vi "SPI_UI.vi"() -> ()   [LabVIEW 2023]
uses:
  ConcreteClasses/ConcreteInstrumentClasses/Multiharp/Multiharp/Types/MH_UIThread_Cmds_T2.ctl
  ConcreteClasses/ConcreteInstrumentClasses/Multiharp/Multiharp/Types/MH_UIThread_Data_T2.ctl
  ConcreteClasses/ConcreteInstrumentClasses/Multiharp/Multiharp/Types/MH_InputChannel.ctl
  ConcreteClasses/ConcreteInstrumentClasses/Multiharp/Multiharp/_lib/PQ/MultiHarp/MH_RefSource.ctl
  ConcreteClasses/ConcreteInstrumentClasses/Multiharp/Multiharp/_lib/PQ/MultiHarp/mhlib_x86_x64_AnyThread.llb/MH_DllPath_global.vi
  <vilib>/Utility/error.llb/DialogType.ctl
  <vilib>/ErrorRing/Error Ring.xnode
  <vilib>/Utility/error.llb/Error Cluster From Error Code.vi
  ConcreteClasses/ConcreteInstrumentClasses/Multiharp/Multiharp/_lib/PQ/MultiHarp/MH_LibVersion_global.vi
  ConcreteClasses/ConcreteInstrumentClasses/Multiharp/Multiharp/_lib/PQ/MultiHarp/MH_MeasMode.ctl
  ConcreteClasses/ConcreteInstrumentClasses/Multiharp/Multiharp/Types/MH_SetInpChanData.ctl
  ConcreteClasses/ConcreteInstrumentClasses/Multiharp/Multiharp/Types/MH_SetInpChanCmds.ctl
  <vilib>/ActorFramework/Message Enqueuer/Message Enqueuer.lvclass
  ConcreteClasses/ConcreteInstrumentClasses/Multiharp/Multiharp/_lib/PQ/MultiHarp/MH_InitInfo.ctl
  typedefs/typedefs.lvlib
panel:
  in  "Init Multiharp":bool
  in  "Refresh(ms)":u32=500
  out "Waveform Chart":dbl[][](graph)
  in  "Monitor Range":i32=40
  in  "Path":path
  in  "FileName 2":string
  in  "Number of Acquisitions":i32=1 min=1 step=1
  out "x*y":dbl
  out "HistoGraph":T1(graph)={0.0, "Resolution"=0.08, "Histograms"=[]}
  in  "Run continuously":enum32{"Running Mode", "Item 1"}(radio) caption="Acquisition"
  in  "Start":bool
  in  "Scale":enum32{"Item 0", "Item 1"}(radio)
  out "CountRates":i32[](graph)
  in  "AllChannels":T2={"Enable"=TRUE, "Offset"=0, "Level"=20, "Edge"=0, "DeadTime"=1000, "UseDeadTime"=FALSE, "SetEnableAllChan"=TRUE, "SetEdgeAllChan"=TRUE, "SetLevelAllChan"=TRUE, "SetOffsetAllChan"=TRUE, "SetUseDTAllChan"=TRUE, "SetDeadTAllChan"=TRUE} {"DeadTime" min=800 max=160000 step=1; "Edge" items=["falling", "rising"]; "Offset" min=-100000 max=100000 step=10; "Level" min=-1200 max=1200 step=1}
  in  "HistoLength":i32(ring)=6 caption="Num Bins" items=["1024", "2048", "4096", "8192", "16384", "32768", "65536"]
  in  "OvlLevel":u32=4294967295 caption="Ovl.Level" min=1 step=1
  in  "StopOvl.":bool=TRUE
  in  "AcqTime":i32=1000 caption="Acqu.           ms" min=1 max=3600000 step=1
  in  "Binning":i32(ring) caption="Resol.            ps" items=["10", "20", "40", "80", "160", "320", "640", "1280", "2560", "5120", "10240", "20480", "40960", "81920", "163840", "327680", "655360", "1310720", "2621440", "5242880", "10485760", "20971520", "41943040"]
  in  "HistoOffset":i32 caption="Offset            ns" min=0 max=100000000 step=1
  in  "Acquire":bool
  in  "stop":bool
  in  "SyncDeadTime":i32=1000 caption="Dead T.   ps" min=800 max=160000 step=1
  in  "UseDeadTime":bool caption="Use DT."
  in  "SyncEdge":i32(ring) caption="Edge" items=["falling", "rising"]
  in  "SyncDivider":i32(ring) caption="Divider" items=["1", "2", "4", "8", "16"]
  in  "SyncOffset":i32 caption="Offset      ps" min=-100000 max=100000 step=10
  in  "SyncLevel":i32=-100 caption="Level      mV" min=-1200 max=1200 step=1
  in  "Channels":T3[](array[typedef])=[{"Name"="Inp.Chan 1", "Enable"=TRUE, "Edge"=0, "Level"=-100, "Offset"=0, "UseDeadTime"=FALSE, "DeadTime"=1000}, {"Name"="Inp.Chan 2", "Enable"=TRUE, "Edge"=0, "Level"=-100, "Offset"=0, "UseDeadTime"=FALSE, "DeadTime"=1000}, {"Name"="Inp.Chan 3", "Enable"=TRUE, "Edge"=0, "Level"=-100, "Offset"=0, "UseDeadTime"=FALSE, "DeadTime"=1000}, {"Name"="Inp.Chan 4", "Enable"=TRUE, "Edge"=0, "Level"=-100, "Offset"=0, "UseDeadTime"=FALSE, "DeadTime"=1000}, {"Name"="Inp.Chan 5", "Enable"=TRUE, "Edge"=0, "Level"=-100, "Offset"=0, "UseDeadTime"=FALSE, "DeadTime"=1000}, {"Name"="Inp.Chan 6", "Enable"=TRUE, "Edge"=0, "Level"=-100, "Offset"=0, "UseDeadTime"=FALSE, "DeadTime"=1000}, {"Name"="Inp.Chan 7", "Enable"=TRUE, "Edge"=0, "Level"=-100, "Offset"=0, "UseDeadTime"=FALSE, "DeadTime"=1000}, {"Name"="Inp.Chan 8", "Enable"=TRUE, "Edge"=0, "Level"=-100, "Offset"=0, "UseDeadTime"=FALSE, "DeadTime"=1000}, {"Name"="Inp.Chan 9", "Enable"=TRUE, "Edge"=0, "Level"=-100, "Offset"=0, "UseDeadTime"=FALSE, "DeadTime"=1000}, {"Name"="Inp.Chan 10", "Enable"=TRUE, "Edge"=0, "Level"=-100, "Offset"=0, "UseDeadTime"=FALSE, "DeadTime"=1000}, {"Name"="Inp.Chan 11", "Enable"=TRUE, "Edge"=0, "Level"=-100, "Offset"=0, "UseDeadTime"=FALSE, "DeadTime"=1000}, {"Name"="Inp.Chan 12", "Enable"=TRUE, "Edge"=0, "Level"=-100, "Offset"=0, "UseDeadTime"=FALSE, "DeadTime"=1000}, {"Name"="Inp.Chan 13", "Enable"=TRUE, "Edge"=0, "Level"=-100, "Offset"=0, "UseDeadTime"=FALSE, "DeadTime"=1000}, {"Name"="Inp.Chan 14", "Enable"=TRUE, "Edge"=0, "Level"=-100, "Offset"=0, "UseDeadTime"=FALSE, "DeadTime"=1000}, {"Name"="Inp.Chan 15", "Enable"=TRUE, "Edge"=0, "Level"=-100, "Offset"=0, "UseDeadTime"=FALSE, "DeadTime"=1000}, {"Name"="Inp.Chan 16", "Enable"=TRUE, "Edge"=0, "Level"=-100, "Offset"=0, "UseDeadTime"=FALSE, "DeadTime"=1000}] {"DeadTime" min=800 max=160000 step=1; "Edge" items=["falling", "rising"]; "Offset" min=-100000 max=100000 step=10; "Level" min=-1200 max=1200 step=1}
  out "SyncRate":string="Sync Rate: 4999950 cps\n"
  out "OverFlow":bool caption="Overflow:"
  out "Status":string="Readout Rate: 8.6 Hz\t\tTotal Counts:\t\tCh. 1: 0 cnts.\t\tCh. 2: 1962112 cnts.\t\tCh. 3: 0 cnts.\t\tCh. 4: 1962112 cnts.\t\tCh. 5: 0 cnts.\t\tCh. 6: 1962112 cnts.\t\tCh. 7: 0 cnts.\t\tCh. 8: 1962112 cnts.\t\tCh. 9: 1962113 cnts.\t\tCh.10: 0 cnts.\t\tCh.11: 1962113 cnts.\t\tCh.12: 0 cnts.\t\tCh.13: 1962113 cnts.\t\tCh.14: 0 cnts.\t\tCh.15: 1962113 cnts.\t\tCh.16: 1962113 cnts.\t\t"
  # "Single Counts"
  # "Coincidences vs time"
  # "Coincidences vs delay"
  # "Acquisition Options"
  # "Acquire Data"
  # "Piezo"
  # "Stage piezo"
  # "Scan"
  # "Jog"
  # "All Channels"
  # "Sync"
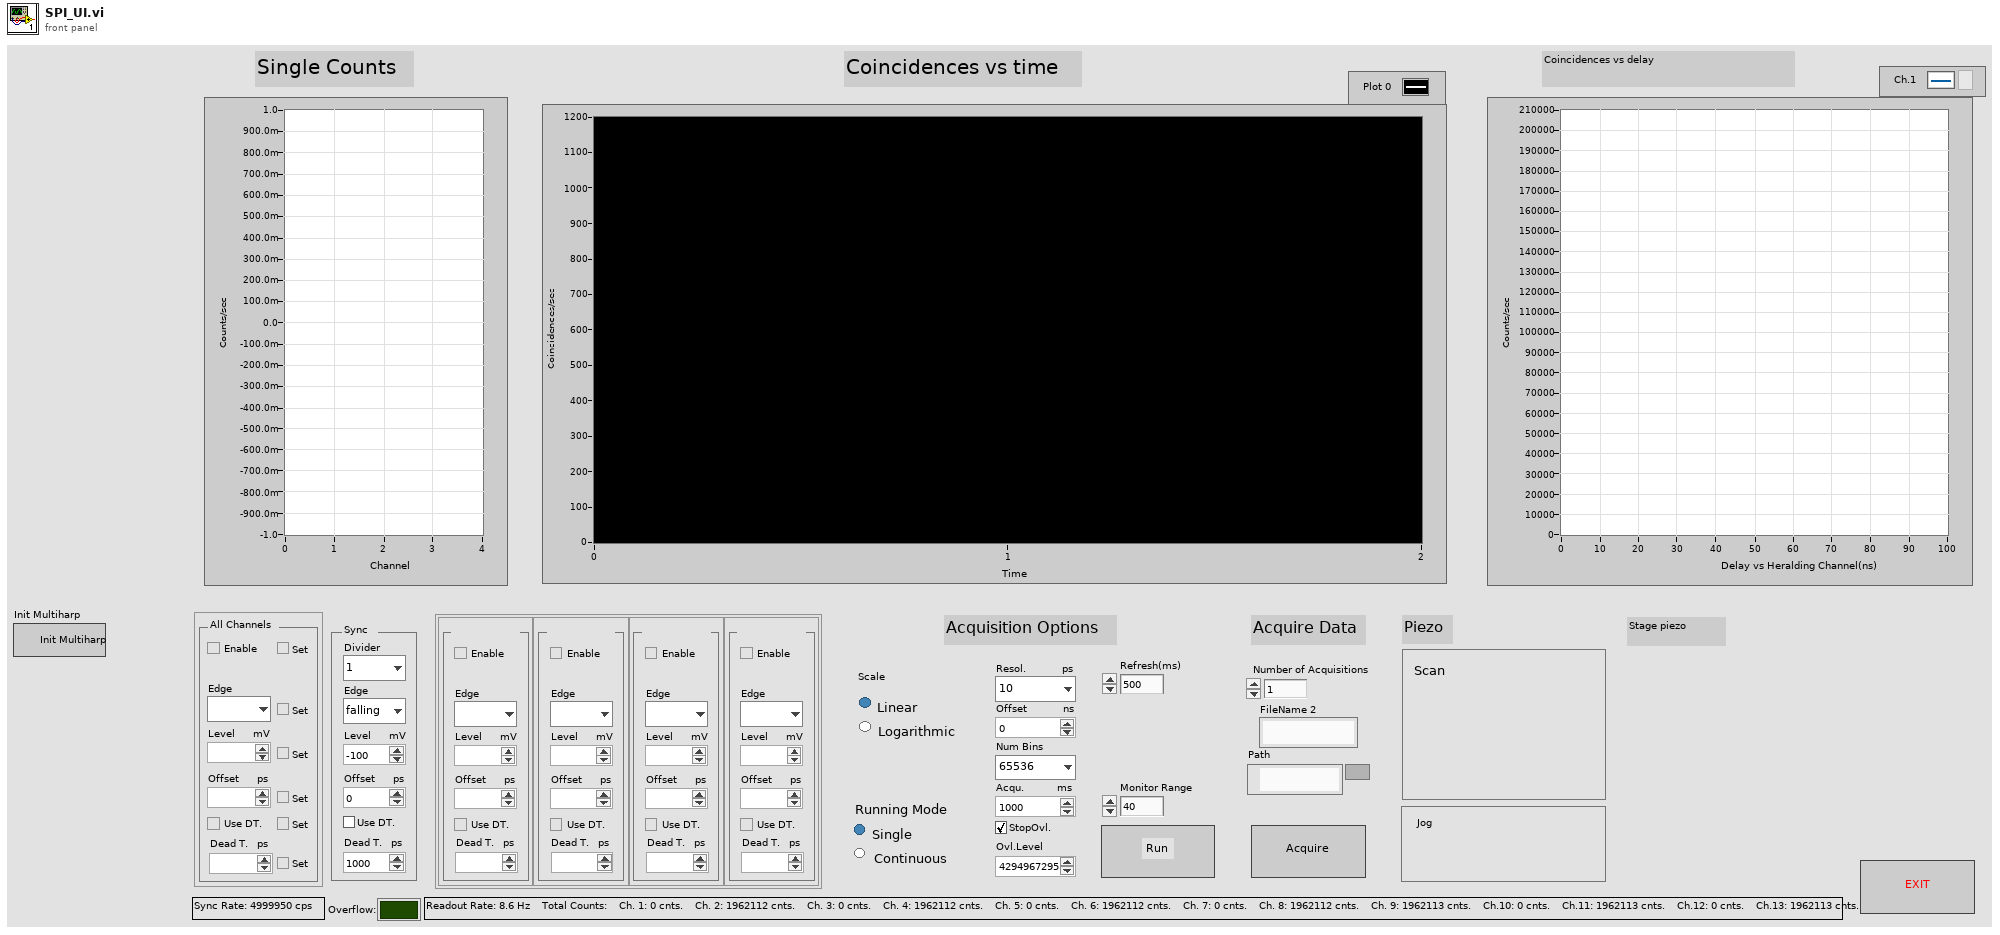
[diagram p1: front panel]
types:
  T1 = cluster{dbl, "Resolution":dbl, "Histograms":u32[][]}
  T2 = cluster{"Enable":bool, "Offset":i32, "Level":i32, "Edge":i32, "DeadTime":i32, "UseDeadTime":bool, "SetEnableAllChan":bool, "SetEdgeAllChan":bool, "SetLevelAllChan":bool, "SetOffsetAllChan":bool, "SetUseDTAllChan":bool, "SetDeadTAllChan":bool}
  T3 = typedef "MH_InputChannel.ctl" = cluster{"Name":string, "Enable":bool, "Edge":i32, "Level":i32, "Offset":i32, "UseDeadTime":bool, "DeadTime":i32}
  T4 = typedef "MH_UIThread_Data_T2.ctl" = cluster{"Init Info":T5, "DevIdx":i32, "SyncDivider":i32, "SyncOffset":i32, "SyncLevel":i32, "Channels":T3[], "CurrentChannels":i32[], "AcqTime":i32, "Binning":i32, "HistoOffset":i32, "HistoLen":i32, "StopOvl.":bool, "OvlLevel":u32, "SyncEdge":i32, "StartMeas":bool, "HistoLength":i32, "Resolution":dbl, "Run cont.":bool, "Status":string, "SyncRate":i32, "BitShift":i32, "HistoAcqTime":dbl, "SyncRateStart":i32, "UseDeadTime":bool, "SyncDeadTime":i32, "SetInpChan":T6[], "max value":u32[], "CoincidenceArray":dbl[][], "Instr Enqueuers":cluster{"MH Enqueuer":refnum<class "Message Enqueuer.lvclass">, "KIM Enqueuer":refnum<class "Message Enqueuer.lvclass">}, "Histo On":bool}
  T5 = typedef "typedefs.lvlib/MH_InitInfo.ctl" = cluster{"Library Version":string, "Serial No.":string, "Model":string, "Partnum":string, "Version":string, "features":i32, "nchannels":i32, "Base Resolution":dbl, "Bin Steps":i32}
  T6 = typedef "MH_SetInpChanData.ctl" = cluster{"Channel":i32, "Cmds":T7[], "Changed":cluster{"Name":bool, "Enable":bool, "Edge":bool, "Level":bool, "Offset":bool, "UseDeadTime":bool, "DeadTime":bool}}
  T7 = typedef "MH_SetInpChanCmds.ctl" = enum16{"SetInpChanEnable", "SetInpChanOffset", "SetInpChanDeadTime", "SetInpChanTrg"}
  T8 = typedef "MH_UIThread_Cmds_T2.ctl" = enum16{"Idle", "Init", "SetInpChan", "SetSyncDivider", "SetSyncTrg", "SetSyncOffset", "SetSyncDeadTime", "SetBinning", "SetHistoOffset", "SetHistoLen", "SetStopOvl", "SetBitShift", "SetHistoAcqTime", "GetRates", "GetAllRates", "StartMeas", "StopMeas", "AbortMeas", "GetResolution", "GetHistos", "GetAllHistos", "ReadFiFo", "WriteStatus", "Resize", "EnableControls", "DisableControls", "Error", "Exit", "Acquire", "InitAcquisition"}
  T9 = enum8{"Enabled", "Disabled", "Disabled and Grayed Out"}
  T10 = typedef "MH_InputChannel2.ctl" = cluster{"Name":string, "Enable":bool, "Edge":i32, "Level":i32, "Offset":i32, "UseDeadTime":bool, "DeadTime":i32}
  T11 = cluster{"[0]":bool, "[1]":bool, "[2]":bool, "[3]":bool, "[4]":bool, "[5]":bool}
  T12 = typedef "MH_MeasMode.ctl" = i32
  T13 = typedef "MH_RefSource.ctl" = enum16{"INTERNAL", "EXTERNAL_10MHZ", "WR_MASTER_GENERIC", "WR_SLAVE_GENERIC", "WR_GRANDM_GENERIC", "EXTN_GPS_PPS", "EXTN_GPS_PPS_UART", "WR_MASTER_MHARP", "WR_SLAVE_MHARP", "WR_GRANDM_MHARP"}
  T14 = cluster{dbl, "Resolution":dbl, "Histogram":u32[][]}
  T15 = typedef "DialogType.ctl" = u16
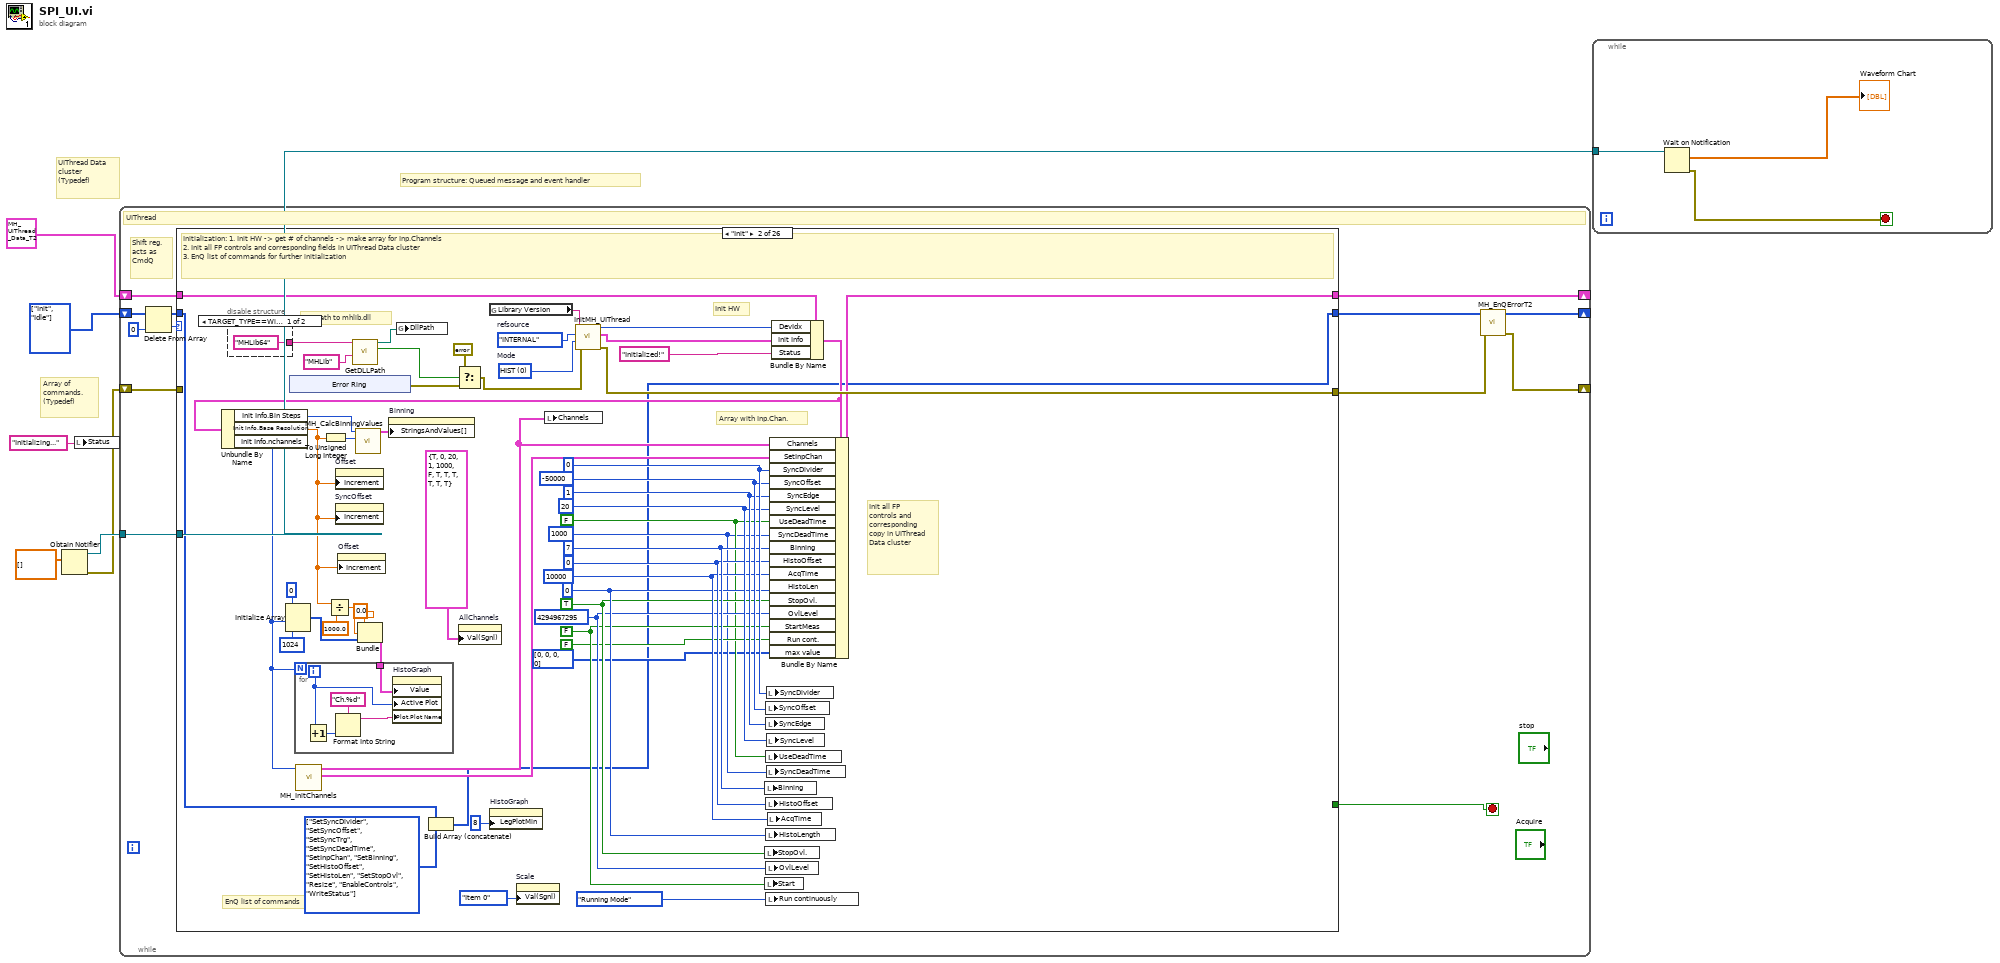
[diagram p0: block diagram]
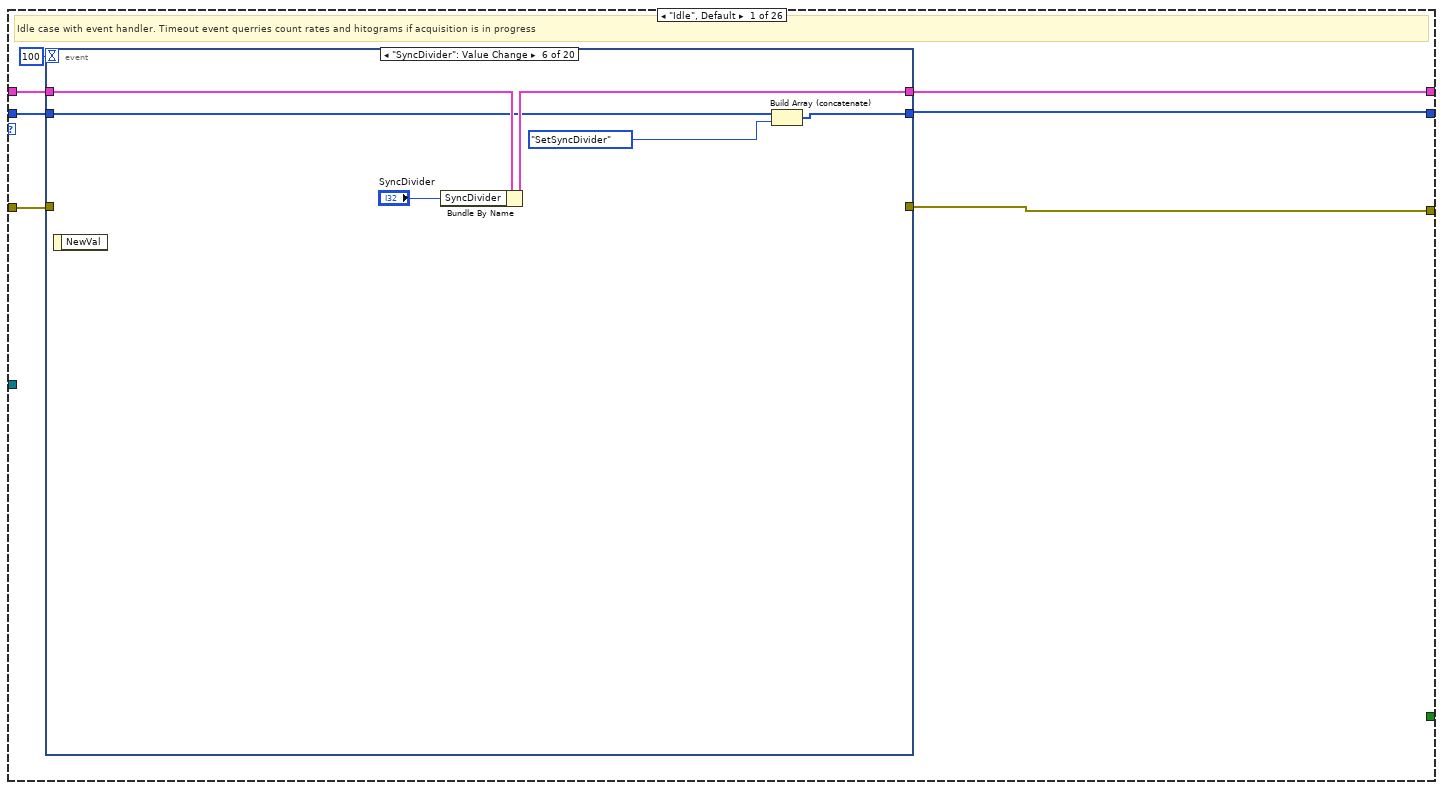
[diagram p2: hidden frame]
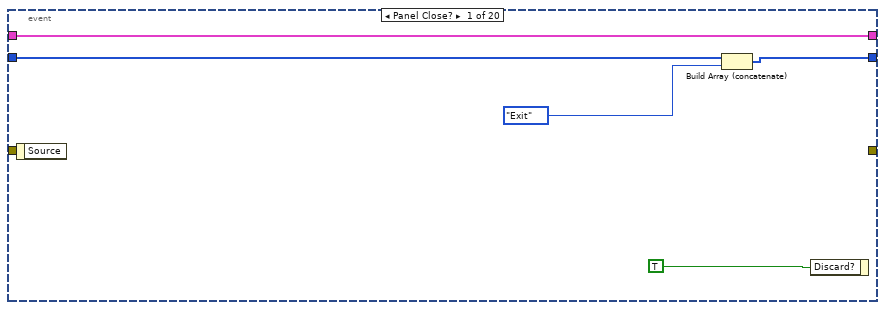
[diagram p3: hidden frame]
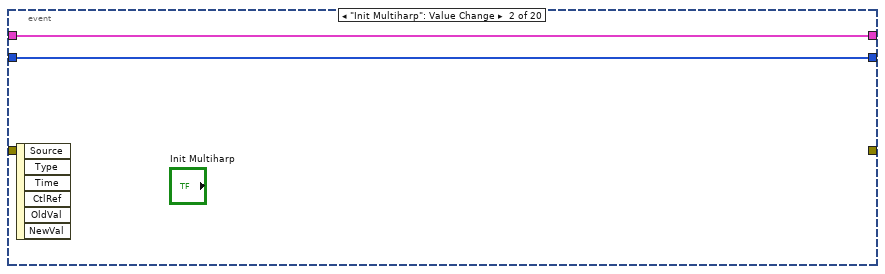
[diagram p4: hidden frame]
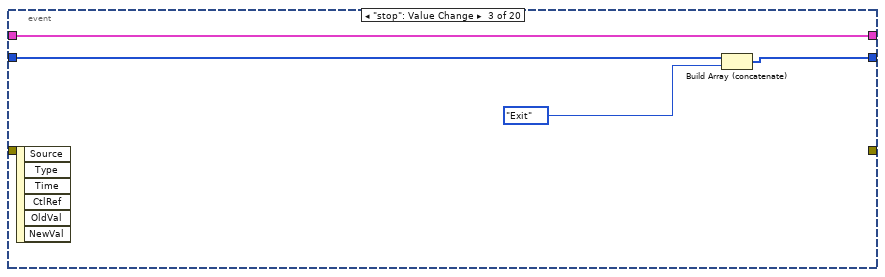
[diagram p5: hidden frame]
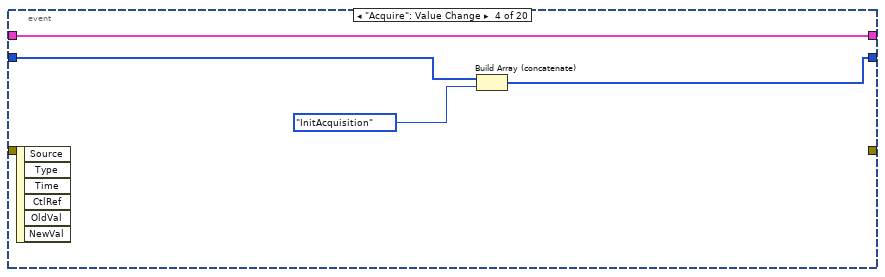
[diagram p6: hidden frame]
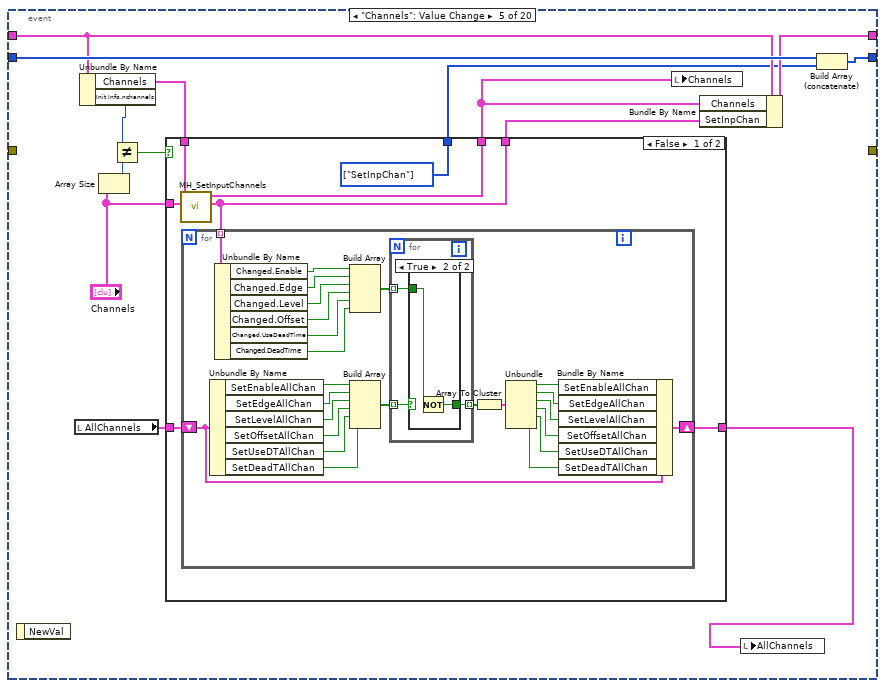
[diagram p7: hidden frame]
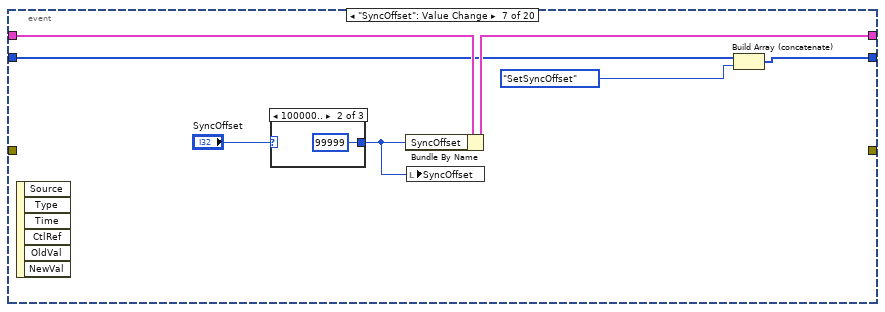
[diagram p10: hidden frame]
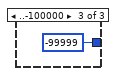
[diagram p12: hidden frame]
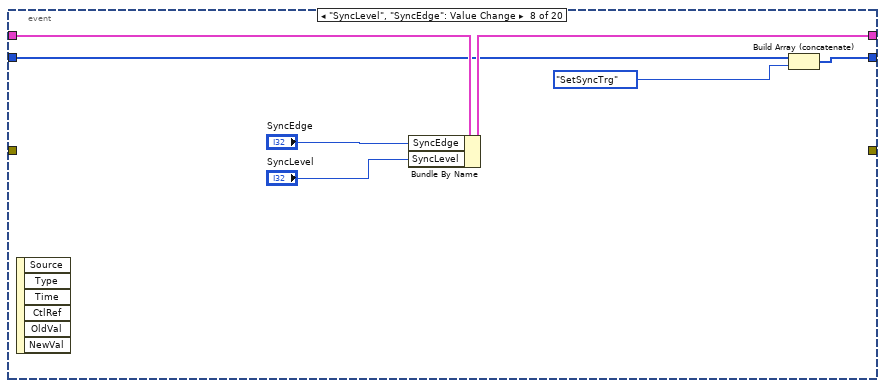
[diagram p13: hidden frame]
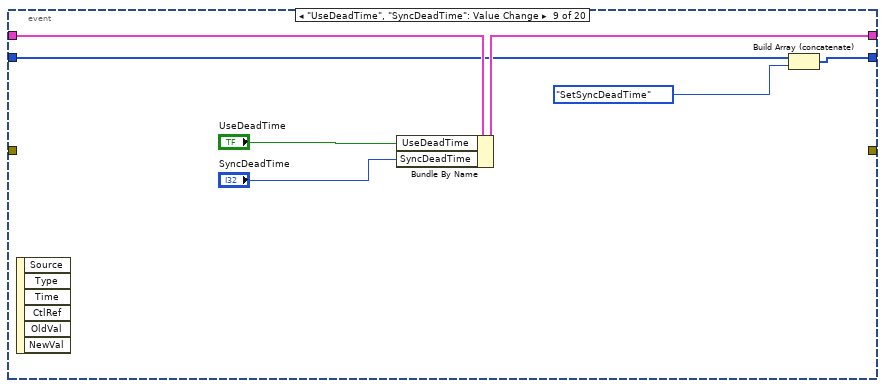
[diagram p14: hidden frame]
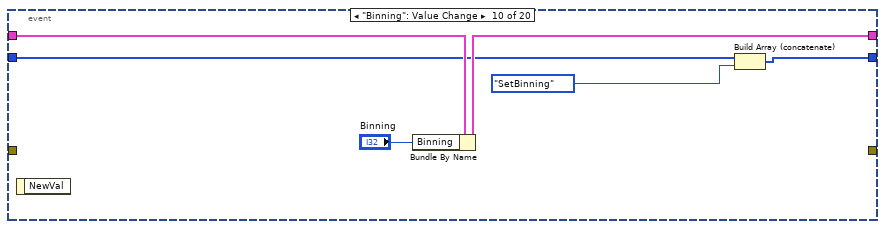
[diagram p15: hidden frame]
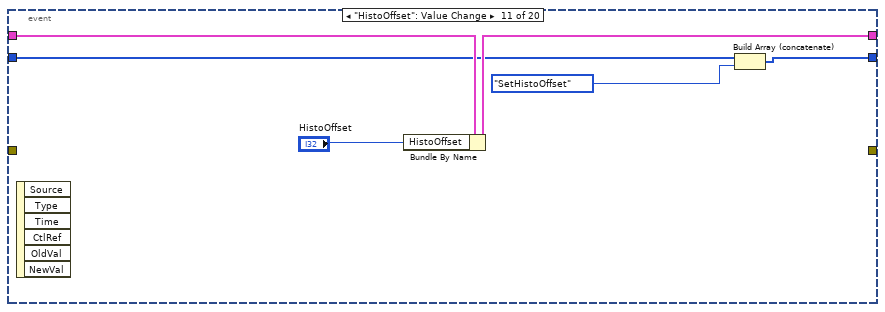
[diagram p16: hidden frame]
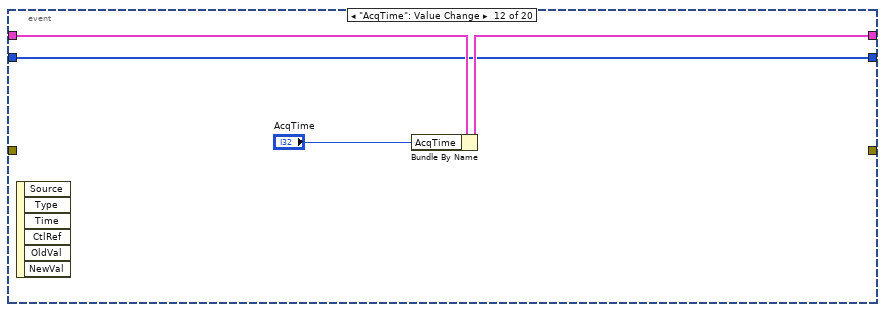
[diagram p17: hidden frame]
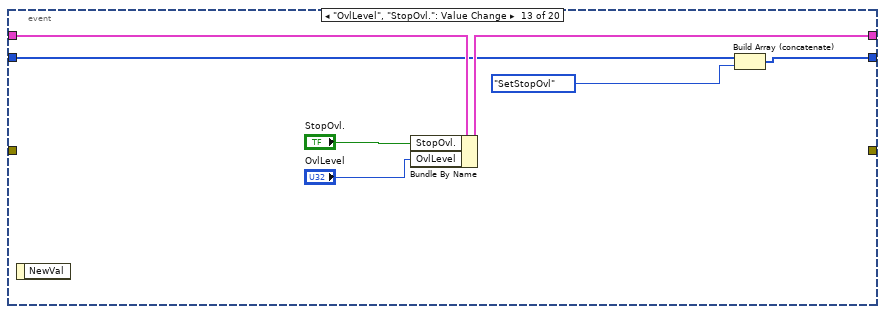
[diagram p18: hidden frame]
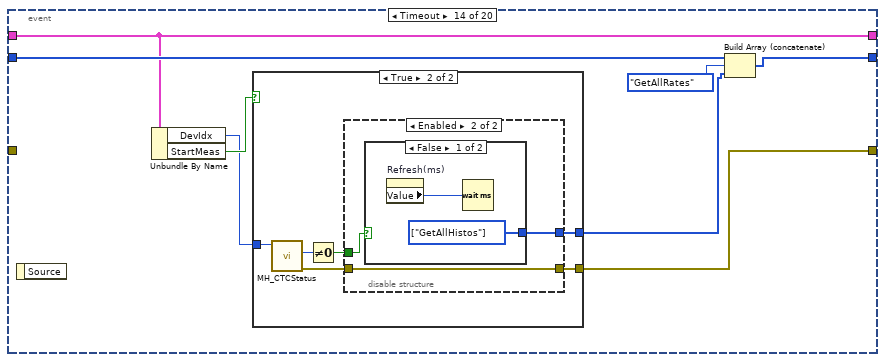
[diagram p19: hidden frame]
diagram:
  w6 = T8[] [enum."Init", enum."Idle"] items=["Idle", "Init", "SetInpChan", "SetSyncDivider", "SetSyncTrg", "SetSyncOffset", "SetSyncDeadTime", "SetBinning", "SetHistoOffset", "SetHistoLen", "SetStopOvl", "SetBitShift", "SetHistoAcqTime", "GetRates", "GetAllRates", "StartMeas", "StopMeas", "AbortMeas", "GetResolution", "GetHistos", "GetAllHistos", "ReadFiFo", "WriteStatus", "Resize", "EnableControls", "DisableControls", "Error", "Exit", "Acquire", "InitAcquisition"]
  # "Array of commands.\n(Typedef)"
  # "Program structure: Queued message and event handler"
  # "UIThread Data cluster\n(Typedef)"
  n1 = Obtain Notifier(notification data type=dbl[][] [] ("element data type")) -> (notifier out=w2:refnum<notifier>, error out=w1:errorcluster)  [unwired: 3 in, 1 out]
  n2 = local write "Status"("Initializing..." ("Status")) -> ()
  n3 = while {
    shift-right: [w9] -> _
    shift-left: w6 -> [w15]
    shift-right: [w18] -> _
    shift-left: T4 {"Init Info"={"Library Version"="", "Serial No."="", "Model"="", "Partnum"="", "Version"="", "features"=0, "nchannels"=0, "Base Resolution"=0.0, "Bin Steps"=0}, "DevIdx"=0, "SyncDivider"=1, "SyncOffset"=0, "SyncLevel"=50, "Channels"=[], "CurrentChannels"=[], "AcqTime"=1, "Binning"=1, "HistoOffset"=1, "HistoLen"=1024, "StopOvl."=FALSE, "OvlLevel"=1024, "SyncEdge"=10, "StartMeas"=FALSE, "HistoLength"=0, "Resolution"=0.0, "Run cont."=FALSE, "Status"="", "SyncRate"=0, "BitShift"=0, "HistoAcqTime"=0.0, "SyncRateStart"=0, "UseDeadTime"=FALSE, "SyncDeadTime"=800, "SetInpChan"=[], "max value"=[], "CoincidenceArray"=[], "Instr Enqueuers"={"MH Enqueuer"=refnum, "KIM Enqueuer"=refnum}, "Histo On"=FALSE} -> [w17]
    shift-right: [w10] -> _
    shift-left: w1 -> [w16]
    tunnel: w2 -> [w8]
    stop <- w19 stop-if-true
    # "Shift reg.\nacts as\nCmdQ"
    # "UIThread"
    n4 = Delete From Array(array=w15, index=0) -> (deleted portion=w13:T8, array with subset deleted=w12:T8[])  [unwired: 1 in]
    n5 = case shown="\"Init\"" w13 {
      tunnel: [_ _ _ _ _ _ _ _ _ _ _ _ _ _ _ _ _ _ _ _ _ _ _ TRUE _ _] -> w19
      tunnel: [w26 w291 w331 w335 w349 w361 w370 w377 w382 w385 w395 w406 w417 w433 w445 w459 w467 w487 w552 w576 w583 w595 w602 w612 w615 w625] -> w18
      tunnel: w17 -> [w25 w296 w331 w335 w349 w361 w370 w377 w382 w386 w395 w406 w417 w434 w446 w460 w468 w488 w552 w576 w583 w595 w602 w612 w615 w625]
      tunnel: [w22 w312 w333 w334 w348 w360 w369 w376 w381 w389 w394 w402 w416 w440 w448 w462 w469 w485 w548 _ _ _ _ w607 w616 w626] -> w11
      tunnel: w16 -> [w20 _ _ _ _ _ _ _ _ _ _ _ _ _ _ _ _ _ _ _ _ _ w603 w610 _ _]
      tunnel: w12 -> [w24 w311 w332 w341 w344 w350 w366 w373 w378 w383 w390 w396 w407 w436 w443 w457 w463 w471 w528 w574 w577 w589 _ w605 w622 w628]
      tunnel: w8 -> [_ _ _ _ _ _ _ _ _ _ _ _ _ _ _ _ _ w482 _ _ _ _ _ w606 _ _]
      tunnel: [w21 w262 w332 w341 w344 w350 w366 w371 w378 w383 w390 w396 w407 w431 w441 w455 w463 w471 w528 w574 w577 w589 w601 w605 w614 w624] -> w7
      frame "Idle", Default {
        # "Idle case with event handler. Timeout event querries count rates and hitograms if acquisition is in progress"
        n6 = event shown="[5] \"SyncDivider\": Value Change" {
          selector: _ -> [_ _ _ _ _ _ _ _ _ _ _ _ _ _ _ _ _ _ _ _]
          dyn-events: _ -> [_ _ _ _ _ _ _ _ _ _ _ _ _ _ _ _ _ _ _ _]
          timeout: 100 -> [_ _ _ _ _ _ _ _ _ _ _ _ _ _ _ _ _ _ _ _]
          tunnel: [w27 w33 w34 w38 w42 w96 w102 w112 w119 w126 w132 w138 w142 w153 w174 w180 w188 w195 w198 w202] -> w21
          tunnel: [w30 w32 w37 w41 w48 w100 w107 w117 w124 w130 w136 w140 w147 w155 w178 w182 w193 w197 w201 w206] -> w26
          tunnel: w25 -> [w30 w32 w37 w41 w50 w101 w108 w118 w125 w131 w137 w141 w148 w155 w179 w183 w194 w197 w201 w207]
          tunnel: w24 -> [w29 w33 w36 w40 w55 w98 w106 w115 w123 w129 w135 w138 w146 w156 w177 w185 w188 w195 w199 w212]
          tunnel: [_ _ _ _ _ _ _ _ _ _ _ _ _ w154 _ _ _ _ _ _] -> w22
          tunnel: w20 -> [_ _ _ _ _ _ _ _ _ _ _ _ _ _ _ _ _ _ _ _]
          event Panel Close? {
            n7 = event-data() -> ()  [unwired: 1 in, 1 out]
            n8 = Build Array (concatenate)(w29, MH_UIThread_Cmds_T2."Exit") -> (w27:T8[])
            n9 = event-data("Discard?"=TRUE) -> ()  [unwired: 1 in, 1 out]
          }
          event "Init Multiharp": Value Change {
            n10 = event-data() -> ()  [unwired: 1 in, 6 out]
          }
          event "stop": Value Change {
            n11 = event-data() -> ()  [unwired: 1 in, 6 out]
            n12 = Build Array (concatenate)(w36, MH_UIThread_Cmds_T2."Exit") -> (w34:T8[])
          }
          event "Acquire": Value Change {
            n13 = event-data() -> ()  [unwired: 1 in, 6 out]
            n14 = Build Array (concatenate)(w40, MH_UIThread_Cmds_T2."InitAcquisition") -> (w38:T8[])
          }
          event "Channels": Value Change {
            n15 = event-data() -> ()  [unwired: 1 in, 1 out]
            n16 = local read "AllChannels"() -> (w44:T2)
            n17 = Unbundle By Name(w50) -> ("Channels"=w51:T3[], "Init Info.nchannels"=w54:i32)
            n18 = Array Size(array="Channels") -> (size(s)=w53:i32)
            n19 = Not Equal?(x=w54, y=w53) -> (x != y?=w52:bool)
            n20 = case shown="False" w52 {
              tunnel: "Channels" -> [w61 _]
              tunnel: [w60 w95] -> w49
              tunnel: w51 -> [w62 w95]
              tunnel: [w58 _] -> w47
              tunnel: [w59 _] -> w45
              tunnel: w44 -> [w57 w94]
              tunnel: [w56 w94] -> w43
              frame False {
                w59 = T8[] [enum."SetInpChan"] items=["Idle", "Init", "SetInpChan", "SetSyncDivider", "SetSyncTrg", "SetSyncOffset", "SetSyncDeadTime", "SetBinning", "SetHistoOffset", "SetHistoLen", "SetStopOvl", "SetBitShift", "SetHistoAcqTime", "GetRates", "GetAllRates", "StartMeas", "StopMeas", "AbortMeas", "GetResolution", "GetHistos", "GetAllHistos", "ReadFiFo", "WriteStatus", "Resize", "EnableControls", "DisableControls", "Error", "Exit", "Acquire", "InitAcquisition"] ("array")
                n21 = call "MH_SetInputChannels.vi"("Channels new"=w61, "Channels old"=w62) -> ("SetInpChan"=w58:T6[], "Channels"=w60:T10[])  [unwired: 8 in]
                n22 = for {
                  tunnel: w58 -> [w87] mode=indexing
                  shift-right: [w69] -> w56
                  shift-left: w57 -> [w71]
                  n23 = Unbundle By Name(w71) -> ("SetEnableAllChan"=w80:bool, "SetEdgeAllChan"=w79:bool, "SetLevelAllChan"=w78:bool, "SetOffsetAllChan"=w77:bool, "SetUseDTAllChan"=w76:bool, "SetDeadTAllChan"=w75:bool)
                  n24 = Unbundle By Name(w87) -> ("Changed.Enable"=w86:bool, "Changed.Edge"=w85:bool, "Changed.Level"=w84:bool, "Changed.Offset"=w83:bool, "Changed.UseDeadTime"=w82:bool, "Changed.DeadTime"=w81:bool)
                  n25 = Build Array(w86, w85, w84, w83, w82, w81) -> (w73:bool[])
                  n26 = Build Array(w80, w79, w78, w77, w76, w75) -> (w74:bool[])
                  n27 = for {
                    tunnel: w74 -> [w90] mode=indexing
                    tunnel: w73 -> [w88] mode=indexing
                    tunnel: [w89] -> w72 mode=indexing
                    n28 = case shown="True" w90 {
                      selector: w90 -> [w91 _]
                      tunnel: [w91 w92] -> w89
                      tunnel: w88 -> [_ w93]
                      frame False {
                      }
                      frame True {
                        n29 = Not(x=w93) -> (.not. x?=w92:bool)
                      }
                    }
                  }
                  n30 = Array To Cluster(array=w72) -> (cluster=w70:T11)
                  n31 = Unbundle(w70) -> ("[0]"=w68:bool, "[1]"=w67:bool, "[2]"=w66:bool, "[3]"=w65:bool, "[4]"=w64:bool, "[5]"=w63:bool)
                  n32 = Bundle By Name(cluster=w71, "SetEnableAllChan"=w68, "SetEdgeAllChan"=w67, "SetLevelAllChan"=w66, "SetOffsetAllChan"=w65, "SetUseDTAllChan"=w64, "SetDeadTAllChan"=w63) -> (w69:T2)
                }
              }
              frame True {
              }
            }
            n33 = local write "Channels"(w49) -> ()
            n34 = Bundle By Name(cluster=w50, "Channels"=w49, "SetInpChan"=w47) -> (w48:T4)
            n35 = local write "AllChannels"(w43) -> ()
            n36 = Build Array (concatenate)(w55, w45) -> (w42:T8[])
          }
          event "SyncDivider": Value Change {
            n37 = event-data() -> ()  [unwired: 1 in, 1 out]
            n38 = Bundle By Name(cluster=w101, "SyncDivider"="SyncDivider") -> (w100:T4)
            n39 = Build Array (concatenate)(w98, MH_UIThread_Cmds_T2."SetSyncDivider") -> (w96:T8[])
          }
          event "SyncOffset": Value Change {
            n40 = event-data() -> ()  [unwired: 1 in, 6 out]
            n41 = case shown="100000.." "SyncOffset" {
              selector: "SyncOffset" -> [w109 _ _]
              tunnel: [w109 99999 ("SyncOffset") -99999 ("SyncOffset")] -> w103
              frame Default {
              }
              frame 100000.. {
              }
              frame ..-100000 {
              }
            }
            n42 = Bundle By Name(cluster=w108, "SyncOffset"=w103) -> (w107:T4)
            n43 = local write "SyncOffset"(w103) -> ()
            n44 = Build Array (concatenate)(w106, MH_UIThread_Cmds_T2."SetSyncOffset") -> (w102:T8[])
          }
          event "SyncLevel", "SyncEdge": Value Change {
            n45 = event-data() -> ()  [unwired: 1 in, 6 out]
            n46 = Bundle By Name(cluster=w118, "SyncEdge"="SyncEdge", "SyncLevel"="SyncLevel") -> (w117:T4)
            n47 = Build Array (concatenate)(w115, MH_UIThread_Cmds_T2."SetSyncTrg") -> (w112:T8[])
          }
          event "UseDeadTime", "SyncDeadTime": Value Change {
            n48 = event-data() -> ()  [unwired: 1 in, 6 out]
            n49 = Bundle By Name(cluster=w125, "UseDeadTime"="UseDeadTime", "SyncDeadTime"="SyncDeadTime") -> (w124:T4)
            n50 = Build Array (concatenate)(w123, MH_UIThread_Cmds_T2."SetSyncDeadTime") -> (w119:T8[])
          }
          event "Binning": Value Change {
            n51 = event-data() -> ()  [unwired: 1 in, 1 out]
            n52 = Bundle By Name(cluster=w131, "Binning"="Binning") -> (w130:T4)
            n53 = Build Array (concatenate)(w129, MH_UIThread_Cmds_T2."SetBinning") -> (w126:T8[])
          }
          event "HistoOffset": Value Change {
            n54 = event-data() -> ()  [unwired: 1 in, 6 out]
            n55 = Bundle By Name(cluster=w137, "HistoOffset"="HistoOffset") -> (w136:T4)
            n56 = Build Array (concatenate)(w135, MH_UIThread_Cmds_T2."SetHistoOffset") -> (w132:T8[])
          }
          event "AcqTime": Value Change {
            n57 = event-data() -> ()  [unwired: 1 in, 6 out]
            n58 = Bundle By Name(cluster=w141, "AcqTime"="AcqTime") -> (w140:T4)
          }
          event "OvlLevel", "StopOvl.": Value Change {
            n59 = event-data() -> ()  [unwired: 1 in, 1 out]
            n60 = Bundle By Name(cluster=w148, "StopOvl."="StopOvl.", "OvlLevel"="OvlLevel") -> (w147:T4)
            n61 = Build Array (concatenate)(w146, MH_UIThread_Cmds_T2."SetStopOvl") -> (w142:T8[])
          }
          event Timeout {
            n62 = event-data() -> ()  [unwired: 1 in, 1 out]
            n63 = Unbundle By Name(w155) -> ("DevIdx"=w150:i32, "StartMeas"=w151:bool)
            n64 = case shown="True" w151 {
              tunnel: w150 -> [_ w162]
              tunnel: [_ w160] -> w149
              tunnel: [_ w157] -> w154
              frame False {
              }
              frame True {
                n65 = call "MH_CTCStatus.vi"("devidx"=w162) -> ("error out"=w158:errorcluster, "ctcstatus"=w161:i32)  [unwired: 8 in, 1 out]
                n66 = Not Equal To 0?(x=w161) -> (x != 0?=w159:bool)
                n67 = disable-structure shown="Enabled" {
                  disable-tunnel: [w167 w169] -> w160
                  disable-tunnel: w159 -> [w165 w170]
                  disable-tunnel: w158 -> [w163 w168]
                  disable-tunnel: [w163 w168] -> w157
                  frame Disabled {
                    w164 = T8[] [enum."GetAllHistos"] items=["Idle", "Init", "SetInpChan", "SetSyncDivider", "SetSyncTrg", "SetSyncOffset", "SetSyncDeadTime", "SetBinning", "SetHistoOffset", "SetHistoLen", "SetStopOvl", "SetBitShift", "SetHistoAcqTime", "GetRates", "GetAllRates", "StartMeas", "StopMeas", "AbortMeas", "GetResolution", "GetHistos", "GetAllHistos", "ReadFiFo", "WriteStatus", "Resize", "EnableControls", "DisableControls", "Error", "Exit", "Acquire", "InitAcquisition"]
                    w166 = T8[] [enum."StopMeas"] items=["Idle", "Init", "SetInpChan", "SetSyncDivider", "SetSyncTrg", "SetSyncOffset", "SetSyncDeadTime", "SetBinning", "SetHistoOffset", "SetHistoLen", "SetStopOvl", "SetBitShift", "SetHistoAcqTime", "GetRates", "GetAllRates", "StartMeas", "StopMeas", "AbortMeas", "GetResolution", "GetHistos", "GetAllHistos", "ReadFiFo", "WriteStatus", "Resize", "EnableControls", "DisableControls", "Error", "Exit", "Acquire", "InitAcquisition"]
                    n68 = Select(t=w166, s=w165, f=w164) -> (s? t:f=w167:T8[])
                  }
                  frame Enabled {
                    n69 = case shown="False" w170 {
                      tunnel: [w172 w173] -> w169
                      frame False {
                        w172 = T8[] [enum."GetAllHistos"] items=["Idle", "Init", "SetInpChan", "SetSyncDivider", "SetSyncTrg", "SetSyncOffset", "SetSyncDeadTime", "SetBinning", "SetHistoOffset", "SetHistoLen", "SetStopOvl", "SetBitShift", "SetHistoAcqTime", "GetRates", "GetAllRates", "StartMeas", "StopMeas", "AbortMeas", "GetResolution", "GetHistos", "GetAllHistos", "ReadFiFo", "WriteStatus", "Resize", "EnableControls", "DisableControls", "Error", "Exit", "Acquire", "InitAcquisition"]
                        n70 = property on="Refresh(ms)" class="DigNum (strict)"() -> ("Value"=w171:u32)  [unwired: 2 in, 2 out]
                        n71 = Wait (ms)(milliseconds to wait=w171) -> ()  [unwired: 1 out]
                      }
                      frame True {
                        w173 = T8[] [enum."StopMeas"] items=["Idle", "Init", "SetInpChan", "SetSyncDivider", "SetSyncTrg", "SetSyncOffset", "SetSyncDeadTime", "SetBinning", "SetHistoOffset", "SetHistoLen", "SetStopOvl", "SetBitShift", "SetHistoAcqTime", "GetRates", "GetAllRates", "StartMeas", "StopMeas", "AbortMeas", "GetResolution", "GetHistos", "GetAllHistos", "ReadFiFo", "WriteStatus", "Resize", "EnableControls", "DisableControls", "Error", "Exit", "Acquire", "InitAcquisition"]
                      }
                    }
                  }
                }
              }
            }
            n72 = Build Array (concatenate)(w156, MH_UIThread_Cmds_T2."GetAllRates", w149) -> (w153:T8[])
          }
          event "HistoLength": Value Change {
            n73 = event-data() -> ()  [unwired: 1 in, 6 out]
            n74 = Bundle By Name(cluster=w179, "HistoLen"="HistoLength") -> (w178:T4)
            n75 = Build Array (concatenate)(w177, MH_UIThread_Cmds_T2."SetHistoLen") -> (w174:T8[])
          }
          event "Start": Value Change {
            n76 = event-data() -> ()  [unwired: 1 in, 1 out]
            n77 = Select(t=MH_UIThread_Cmds_T2."StartMeas", s="Start", f=MH_UIThread_Cmds_T2."AbortMeas") -> (s? t:f=w184:T8)
            n78 = Bundle By Name(cluster=w183, "StartMeas"="Start") -> (w182:T4)
            n79 = Build Array (concatenate)(w185, w184) -> (w180:T8[])
          }
          event "Run continuously": Value Change {
            n80 = event-data() -> ()  [unwired: 1 in, 1 out]
            n81 = Number To Boolean Array(number="Run continuously") -> (Boolean array=w191:bool[])
            n82 = Delete From Array(array=w191, index=0) -> (deleted portion=w189:bool)  [unwired: 1 in, 1 out]
            n83 = Bundle By Name(cluster=w194, "Run cont."=w189) -> (w193:T4)
          }
          event "Scale": Value Change {
            n84 = event-data() -> ()  [unwired: 1 in, 1 out]
            n85 = property on="HistoGraph" class="WFGraph (strict)"("YScale.Mapping Mode"="Scale") -> ()  [unwired: 2 in, 2 out]
          }
          event Panel Resize {
            n86 = event-data() -> ()  [unwired: 1 in, 1 out]
            n87 = Build Array (concatenate)(w199, MH_UIThread_Cmds_T2."Resize") -> (w198:T8[])
          }
          event "AllChannels": Value Change {
            w204 = T8[] [enum."SetInpChan"] items=["Idle", "Init", "SetInpChan", "SetSyncDivider", "SetSyncTrg", "SetSyncOffset", "SetSyncDeadTime", "SetBinning", "SetHistoOffset", "SetHistoLen", "SetStopOvl", "SetBitShift", "SetHistoAcqTime", "GetRates", "GetAllRates", "StartMeas", "StopMeas", "AbortMeas", "GetResolution", "GetHistos", "GetAllHistos", "ReadFiFo", "WriteStatus", "Resize", "EnableControls", "DisableControls", "Error", "Exit", "Acquire", "InitAcquisition"] ("array")
            n88 = event-data() -> ()  [unwired: 1 in, 1 out]
            n89 = local read "Channels"() -> (w211:T3[])
            n90 = for {
              tunnel: w211 -> [w215] mode=indexing
              tunnel: "AllChannels" -> [w214]
              tunnel: [w213] -> w209 mode=indexing
              n91 = Unbundle By Name(w214) -> ("SetEnableAllChan"=w216:bool, "SetEdgeAllChan"=w217:bool, "SetLevelAllChan"=w218:bool, "SetOffsetAllChan"=w219:bool, "SetUseDTAllChan"=w220:bool, "SetDeadTAllChan"=w221:bool)
              n92 = Build Array(w216, w217, w218, w219, w220, w221) -> (w222:bool[])
              n93 = for {
                tunnel: w222 -> [w227] mode=indexing
                shift-right: [w224] -> w213
                shift-left: w215 -> [w225]
                tunnel: w214 -> [w223]
                i -> [w226]
                n94 = case shown="True" w227 {
                  tunnel: w226 -> [_ w232]
                  tunnel: w223 -> [_ w231]
                  tunnel: w225 -> [w228 w230]
                  tunnel: [w228 w229] -> w224
                  frame False {
                  }
                  frame True {
                    n95 = case shown="Default" w232 {
                      tunnel: w231 -> [w236 w240 w244 w249 w256 w260 _]
                      tunnel: w230 -> [w235 w239 w243 w248 w255 w259 w261]
                      tunnel: [w233 w237 w241 w247 w253 w257 w261] -> w229
                      frame 0 {
                        n96 = Unbundle By Name(w236) -> ("Enable"=w234:bool)
                        n97 = Bundle By Name(cluster=w235, "Enable"=w234) -> (w233:T3)
                      }
                      frame 1 {
                        n98 = Unbundle By Name(w240) -> ("Edge"=w238:i32)
                        n99 = Bundle By Name(cluster=w239, "Edge"=w238) -> (w237:T3)
                      }
                      frame 2 {
                        n100 = Unbundle By Name(w244) -> ("Level"=w242:i32)
                        n101 = Bundle By Name(cluster=w243, "Level"=w242) -> (w241:T3)
                      }
                      frame 3 {
                        n102 = Unbundle By Name(w249) -> ("Offset"=w246:i32)
                        n103 = case shown="100000.." w246 {
                          selector: w246 -> [w250 _ _]
                          tunnel: [w250 99999 ("SyncOffset") -99999 ("SyncOffset")] -> w245
                          frame Default {
                          }
                          frame 100000.. {
                          }
                          frame ..-100000 {
                          }
                        }
                        n104 = Bundle By Name(cluster=w248, "Offset"=w245) -> (w247:T3)
                      }
                      frame 4 {
                        n105 = Unbundle By Name(w256) -> ("UseDeadTime"=w254:bool)
                        n106 = Bundle By Name(cluster=w255, "UseDeadTime"=w254) -> (w253:T3)
                      }
                      frame 5 {
                        n107 = Unbundle By Name(w260) -> ("DeadTime"=w258:i32)
                        n108 = Bundle By Name(cluster=w259, "DeadTime"=w258) -> (w257:T3)
                      }
                      frame Default {
                      }
                    }
                  }
                }
              }
            }
            n109 = Build Array (concatenate)(w212, w204) -> (w202:T8[])
            n110 = Unbundle By Name(w207) -> ("Channels"=w208:T3[])
            n111 = call "MH_SetInputChannels.vi"("Channels new"=w209, "Channels old"=w208) -> ("SetInpChan"=w205:T6[], "Channels"=w203:T10[])  [unwired: 8 in]
            n112 = local write "Channels"(w203) -> ()
            n113 = Bundle By Name(cluster=w207, "Channels"=w203, "SetInpChan"=w205) -> (w206:T4)
          }
        }
      }
      frame "Init" {
        w273 = 1000 ("SyncDeadTime")
        w274 = FALSE ("UseDeadTime")
        w276 = T12 0 items=["HIST"=0, "T2"=2, "T3"=3]  # Mode
        w285 = MH_RefSource."INTERNAL"  # refsource
        w299 = FALSE ("StartMeas")
        w300 = u32 4294967295 ("OvlLevel")
        w301 = TRUE ("StopOvl.")
        w302 = 0 ("HistoLen")
        w303 = 10000 ("AcqTime")
        w304 = 0 ("HistoOffset")
        w305 = 7 ("Binning")
        w306 = 20 ("SyncLevel")
        w307 = 1 ("SyncZeroX")
        w308 = -50000 ("SyncOffset")
        w309 = 0 ("SyncDivider")
        w310 = T8[] [enum."SetSyncDivider", enum."SetSyncOffset", enum."SetSyncTrg", enum."SetSyncDeadTime", enum."SetInpChan", enum."SetBinning", enum."SetHistoOffset", enum."SetHistoLen", enum."SetStopOvl", enum."Resize", enum."EnableControls", enum."WriteStatus"] items=["Idle", "Init", "SetInpChan", "SetSyncDivider", "SetSyncTrg", "SetSyncOffset", "SetSyncDeadTime", "SetBinning", "SetHistoOffset", "SetHistoLen", "SetStopOvl", "SetBitShift", "SetHistoAcqTime", "GetRates", "GetAllRates", "StartMeas", "StopMeas", "AbortMeas", "GetResolution", "GetHistos", "GetAllHistos", "ReadFiFo", "WriteStatus", "Resize", "EnableControls", "DisableControls", "Error", "Exit", "Acquire", "InitAcquisition"]
        # "Init HW"
        # "Set path to mhlib.dll"
        # "Init all FP controls and corresponding copy in UIThread Data cluster"
        # "EnQ list of commands"
        # "Array with Inp.Chan."
        # "Initialization: 1. Init HW -> get # of channels -> make array for Inp.Channels\n2. Init all FP controls and corresponding fields in UIThread Data cluster\n3. EnQ list of commands for further initialization"
        n114 = disable-structure shown="TARGET_TYPE==Windows, Default" {
          disable-tunnel: ["MHLib64" ("name or relative path") "MHLib" ("name or relative path")] -> w275
          frame condition #0 (active) {
          }
          frame condition #1 {
          }
        }
        n115 = xnode "Error Ring"() -> ("error out"=w286:errorcluster)
        n116 = call "GetDLLPath.vi"("DllName_32bit"="MHLib" ("name or relative path"), "DllName_64bit"=w275) -> ("file exists?"=w288:bool, "DLLPath"=w289:path)  [unwired: 8 in]
        n117 = global write "MH_DllPath_global.vi" "DllPath"(w289) -> ()
        n118 = Build Array (concatenate)(w311, w310) -> (w262:T8[])
        n119 = Select(t=errorcluster {"status"=FALSE, "code"=0, "source"=""} ("error IO"), s=w288, f=w286) -> (s? t:f=w292:errorcluster)
        n120 = property on="AllChannels" class="Clust (strict)"("Val(Sgnl)"=T2 {"Enable"=TRUE, "Offset"=0, "Level"=20, "Edge"=1, "DeadTime"=1000, "UseDeadTime"=FALSE, "SetEnableAllChan"=TRUE, "SetEdgeAllChan"=TRUE, "SetLevelAllChan"=TRUE, "SetOffsetAllChan"=TRUE, "SetUseDTAllChan"=TRUE, "SetDeadTAllChan"=TRUE} ("AllChannels")) -> ()  [unwired: 2 in, 2 out]
        n121 = global read "MH_LibVersion_global.vi" "Library Version"() -> (w284:string)
        n122 = property on="HistoGraph" class="WFGraph (strict)"("LegPlotMin"=u32 8 ("Legend:Plot Minimum")) -> ()  [unwired: 2 in, 2 out]
        n123 = property on="Scale" class="RadioBtnsControl (strict)"("Val(Sgnl)"=enum32{"Item 0", "Item 1"}."Item 0" ("Value (Signaling)")) -> ()  [unwired: 2 in, 2 out]
        n124 = call "InitMH_UIThread.vi"("error in (no error)"=w292, "Mode"=w276, "refsource"=w285, "Library Version"=w284) -> ("error out"=w312:errorcluster, "Init Info"=w314:T5, "DevIdx"=w313:i32)  [unwired: 5 in]
        n125 = local write "Binning"(w305) -> ()
        n126 = local write "StopOvl."(w301) -> ()
        n127 = local write "Start"(w299) -> ()
        n128 = local write "SyncOffset"(w308) -> ()
        n129 = local write "SyncEdge"(w307) -> ()
        n130 = local write "UseDeadTime"(w274) -> ()
        n131 = local write "HistoOffset"(w304) -> ()
        n132 = local write "HistoLength"(w302) -> ()
        n133 = local write "OvlLevel"(w300) -> ()
        n134 = local write "Run continuously"(enum32{"Running Mode", "Item 1"}."Running Mode" ("Run continuously")) -> ()
        n135 = local write "SyncDivider"(w309) -> ()
        n136 = local write "SyncLevel"(w306) -> ()
        n137 = local write "SyncDeadTime"(w273) -> ()
        n138 = local write "AcqTime"(w303) -> ()
        n139 = Bundle By Name(cluster=w296, "DevIdx"=w313, "Init Info"=w314, "Status"="Initialized!") -> (w295:T4)
        n140 = Unbundle By Name(w295) -> ("Init Info.Bin Steps"=w294:i32, "Init Info.Base Resolution"=w266:dbl, "Init Info.nchannels"=w271:i32)
        n141 = Initialize Array(u32 0, w271, 1024 ("dimension size")) -> (w278:u32[][])
        n142 = call "MH_InitChannels.vi"("nchannels"=w271) -> ("SetInpChan"=w269:T6[], "Channels"=w270:T10[])  [unwired: 9 in]
        n143 = To Unsigned Long Integer(number=w266) -> (unsigned 32bit integer=w267:u32)
        n144 = Divide(x=w266, y=1000.0) -> (x/y=w279:dbl)
        n145 = property on="Offset" class="DigNum (strict)"("Increment"=w266) -> ()  [unwired: 2 in, 2 out]
        n146 = property on="SyncOffset" class="DigNum (strict)"("Increment"=w266) -> ()  [unwired: 2 in, 2 out]
        n147 = property on="Offset" class="DigNum (strict)"("Increment"=w266) -> ()  [unwired: 2 in, 2 out]
        n148 = call "MH_CalcBinningValues.vi"("BaseResolution"=w267, "Bin Steps"=w294) -> ("BinningValues"=w298:cluster{"String":string, "Value":i32}[])  [unwired: 9 in]
        n149 = Bundle(0.0, w279, w278) -> (w272:cluster{dbl, dbl, u32[][]})  [unwired: 1 in]
        n150 = for {
          N: w271 -> [_]
          tunnel: w272 -> [w322]
          i -> [w324]
          n151 = Increment(x=w324) -> (x+1=w323:i32)
          n152 = Format Into String(format string="Ch.%d", w323) -> (resulting string=w325:string)  [unwired: 2 in, 1 out]
          n153 = property on="HistoGraph" class="WFGraph (strict)"("Value"=w322, "Active Plot"=w324, "Plot.Plot Name"=w325) -> ()  [unwired: 2 in, 2 out]
        }
        n154 = property on="Binning" class="Ring (strict)"("StringsAndValues[]"=w298) -> ()  [unwired: 2 in, 2 out]
        n155 = local write "Channels"(w270) -> ()
        n156 = Bundle By Name(cluster=w295, "Channels"=w270, "SetInpChan"=w269, "SyncDivider"=w309, "SyncOffset"=w308, "SyncEdge"=w307, "SyncLevel"=w306, "UseDeadTime"=w274, "SyncDeadTime"=w273, "Binning"=w305, "HistoOffset"=w304, "AcqTime"=w303, "HistoLen"=w302, "StopOvl."=w301, "OvlLevel"=w300, "StartMeas"=w299, "Run cont."=FALSE, "max value"=u32[] [0, 0, 0, 0]) -> (w291:T4)
      }
      frame "SetInpChan" {
        n157 = Unbundle By Name(w331) -> ("DevIdx"=w330:i32, "Init Info.features"=w329:i32, "SetInpChan"=w328:T6[], "Channels"=w327:T3[])
        n158 = call "SetInputChannels.vi"("Channels"=w327, "SetInpChan"=w328, "features"=w329, 11:w330) -> ("error out"=w333:errorcluster)  [unwired: 7 in]
      }
      frame "SetSyncDivider" {
        n159 = Unbundle By Name(w335) -> ("DevIdx"=w336:i32, "SyncDivider"=w338:i32)
        n160 = Power Of 2(x=w338) -> (2^x=w339:dbl)
        n161 = To Long Integer(number=w339) -> (32bit integer=w340:i32)
        n162 = call "MH_SetSyncDiv.vi"("SyncDivider"=w340, "devidx"=w336) -> ("error out"=w337:errorcluster)  [unwired: 8 in, 1 out]
        n163 = flat-sequence {
          tunnel: w337 -> [w342]
          tunnel: [w342] -> w334
          frame #0 {
            n164 = Wait (ms)(milliseconds to wait=u32 100) -> ()  [unwired: 1 out]
          }
        }
      }
      frame "SetSyncTrg" {
        n165 = Unbundle By Name(w349) -> ("DevIdx"=w347:i32, "SyncLevel"=w345:i32, "SyncEdge"=w346:i32)
        n166 = call "MH_SetSyncEdgeTrg.vi"("edge"=w346, "level"=w345, "devidx"=w347) -> ("error out"=w348:errorcluster)  [unwired: 7 in, 1 out]
      }
      frame "SetSyncDeadTime" {
        w353 = 32  # FEATURE_PROG_TD
        n167 = Unbundle By Name(w361) -> ("DevIdx"=w359:i32, "UseDeadTime"=w357:bool, "SyncDeadTime"=w358:i32, "Init Info.features"=w352:i32)
        n168 = Boolean To (0,1)(Boolean=w357) -> (0, 1=w356:i16)
        n169 = And(x=w352, y=w353) -> (x .and. y?=w354:i32)
        n170 = To Long Integer(number=w356) -> (32bit integer=w355:i32)
        n171 = Not Equal To 0?(x=w354) -> (x != 0?=w351:bool)
        n172 = case shown="True" w351 {
          tunnel: [_ w365] -> w360
          tunnel: w359 -> [_ w364]
          tunnel: w358 -> [_ w363]
          tunnel: w355 -> [_ w362]
          frame False {
          }
          frame True {
            n173 = call "MH_SetSyncDeadTime.vi"("deadtime"=w363, "on"=w362, "devidx"=w364) -> ("error out"=w365:errorcluster)  [unwired: 7 in, 1 out]
          }
        }
      }
      frame "SetSyncOffset" {
        n174 = Unbundle By Name(w370) -> ("DevIdx"=w368:i32, "SyncOffset"=w367:i32)
        n175 = call "MH_SetSyncChannelOffset.vi"("Offset"=w367, "devidx"=w368) -> ("error out"=w369:errorcluster)  [unwired: 8 in, 1 out]
      }
      frame "SetBinning" {
        # "When binning is changed the new resolution is querried"
        n176 = Unbundle By Name(w377) -> ("DevIdx"=w375:i32, "Binning"=w374:i32)
        n177 = call "MH_SetBinning.vi"("Binning"=w374, "devidx"=w375) -> ("error out"=w376:errorcluster)  [unwired: 8 in, 1 out]
        n178 = Build Array (concatenate)(MH_UIThread_Cmds_T2."GetResolution", w373) -> (w371:T8[])
      }
      frame "SetHistoOffset" {
        n179 = Unbundle By Name(w382) -> ("DevIdx"=w380:i32, "HistoOffset"=w379:i32)
        n180 = call "MH_SetOffset.vi"("Offset"=w379, "devidx"=w380) -> ("error out"=w381:errorcluster)  [unwired: 8 in, 1 out]
      }
      frame "SetHistoLen" {
        n181 = Unbundle By Name(w386) -> ("DevIdx"=w388:i32, "HistoLen"=w387:i32)
        n182 = call "MH_SetHistoLen.vi"("lencode"=w387, "devidx"=w388) -> ("error out"=w389:errorcluster, "actuallen"=w384:i32)  [unwired: 7 in, 1 out]
        n183 = Bundle By Name(cluster=w386, "HistoLength"=w384) -> (w385:T4)
      }
      frame "SetStopOvl" {
        n184 = Unbundle By Name(w395) -> ("DevIdx"=w393:i32, "StopOvl."=w392:bool, "OvlLevel"=w391:u32)
        n185 = call "MH_SetStopOverflow.vi"("stopcount"=w391, "StopOnOverflow"=w392, "devidx"=w393) -> ("error out"=w394:errorcluster)  [unwired: 7 in, 1 out]
      }
      frame "GetAllRates" {
        # "An alternative to GetRates"
        n186 = Unbundle By Name(w406) -> ("DevIdx"=w403:i32, "Init Info.nchannels"=w400:i32)
        n187 = call "MH_AllocateCntRateBuffer.vi"("NumChan"=w400) -> ("Buffer"=w401:i32[])  [unwired: 10 in]
        n188 = call "MH_GetAllCountRates.vi"("cntrates_buf"=w401, "devidx"=w403) -> ("error out"=w402:errorcluster, "cntrates"=w398:i32[], "syncrate"=w399:i32)  [unwired: 6 in, 1 out]
        n189 = Build Array (concatenate)(w399, w398) -> (→"CountRates":i32[])
        n190 = Format Into String(format string="Sync Rate: %d cps\n", w399) -> (resulting string=→"SyncRate":string)  [unwired: 2 in, 1 out]
      }
      frame "GetRates" {
        # "An alternative to GetAllRates"
        n191 = Unbundle By Name(w417) -> ("Init Info.nchannels"=w412:i32, "Channels"=w414:T3[], "DevIdx"=w413:i32)
        n192 = call "MH_GetSyncRate.vi"("devidx"=w413) -> ("error out"=w410:errorcluster, "syncrate"=w409:i32)  [unwired: 8 in, 1 out]
        n193 = Format Into String(format string="Sync Rate: %d cps\n", w409) -> (resulting string=w411:string)  [unwired: 2 in, 1 out]
        n194 = for {
          N: w412 -> [_]
          tunnel: w413 -> [w423]
          tunnel: [w420] -> w408 mode=indexing
          shift-right: [w422] -> w416
          shift-left: w410 -> [w424]
          tunnel: w414 -> [w419] mode=indexing
          i -> [w421]
          n195 = Unbundle By Name(w419) -> ("Enable"=w418:bool)
          n196 = case shown="True" w418 {
            tunnel: w424 -> [w425 w430]
            tunnel: w423 -> [_ w429]
            tunnel: [w425 w428] -> w422
            tunnel: w421 -> [_ w427]
            tunnel: [_ w426] -> w420
            frame False {
            }
            frame True {
              n197 = call "MH_GetCountRate.vi"("error in (no error)"=w430, "Channel"=w427, "devidx"=w429) -> ("error out"=w428:errorcluster, "rate"=w426:i32)  [unwired: 6 in, 1 out]
            }
          }
        }
        n198 = local write "CountRates"(w408) -> ()
        n199 = local write "SyncRate"(w411) -> ()
      }
      frame "StartMeas" {
        n200 = Unbundle By Name(w434) -> ("AcqTime"=w437:i32, "DevIdx"=w438:i32)
        n201 = call "MH_ClearHistMem.vi"("devidx"=w438) -> ("error out"=w439:errorcluster)  [unwired: 9 in, 1 out]
        n202 = call "MH_StartMeas.vi"("error in (no error)"=w439, "tacq"=w437, "devidx"=w438) -> ("error out"=w440:errorcluster)  [unwired: 7 in, 1 out]
        n203 = Build Array (concatenate)(w436, MH_UIThread_Cmds_T2."GetAllHistos") -> (w431:T8[])
        n204 = Bundle By Name(cluster=w434, "max value"=u32[] [0, 0, 0, 0]) -> (w433:T4)
      }
      frame "StopMeas" {
        n205 = Unbundle By Name(w446) -> ("Run cont."=w442:bool, "DevIdx"=w447:i32)
        n206 = call "MH_StopMeas.vi"("devidx"=w447) -> ("error out"=w448:errorcluster)  [unwired: 9 in, 1 out]
        n207 = case shown="False" w442 {
          tunnel: w446 -> [w452 w454]
          tunnel: [w451 w454] -> w445
          tunnel: [w449 w453] -> w444
          frame False {
            w449 = T8[] [enum."GetAllHistos"] items=["Idle", "Init", "SetInpChan", "SetSyncDivider", "SetSyncTrg", "SetSyncOffset", "SetSyncDeadTime", "SetBinning", "SetHistoOffset", "SetHistoLen", "SetStopOvl", "SetBitShift", "SetHistoAcqTime", "GetRates", "GetAllRates", "StartMeas", "StopMeas", "AbortMeas", "GetResolution", "GetHistos", "GetAllHistos", "ReadFiFo", "WriteStatus", "Resize", "EnableControls", "DisableControls", "Error", "Exit", "Acquire", "InitAcquisition"]
            w450 = FALSE ("StartMeas")
            n208 = Bundle By Name(cluster=w452, "StartMeas"=w450) -> (w451:T4)
            n209 = local write "Start"(w450) -> ()
          }
          frame True {
            w453 = T8[] [enum."GetAllHistos", enum."StartMeas"] items=["Idle", "Init", "SetInpChan", "SetSyncDivider", "SetSyncTrg", "SetSyncOffset", "SetSyncDeadTime", "SetBinning", "SetHistoOffset", "SetHistoLen", "SetStopOvl", "SetBitShift", "SetHistoAcqTime", "GetRates", "GetAllRates", "StartMeas", "StopMeas", "AbortMeas", "GetResolution", "GetHistos", "GetAllHistos", "ReadFiFo", "WriteStatus", "Resize", "EnableControls", "DisableControls", "Error", "Exit", "Acquire", "InitAcquisition"]
          }
        }
        n210 = Build Array (concatenate)(w443, w444) -> (w441:T8[])
      }
      frame "AbortMeas" {
        w458 = T8[] [enum."GetAllHistos"] items=["Idle", "Init", "SetInpChan", "SetSyncDivider", "SetSyncTrg", "SetSyncOffset", "SetSyncDeadTime", "SetBinning", "SetHistoOffset", "SetHistoLen", "SetStopOvl", "SetBitShift", "SetHistoAcqTime", "GetRates", "GetAllRates", "StartMeas", "StopMeas", "AbortMeas", "GetResolution", "GetHistos", "GetAllHistos", "ReadFiFo", "WriteStatus", "Resize", "EnableControls", "DisableControls", "Error", "Exit", "Acquire", "InitAcquisition"]
        w456 = FALSE ("StartMeas")
        n211 = Unbundle By Name(w460) -> ("DevIdx"=w461:i32)
        n212 = call "MH_StopMeas.vi"("devidx"=w461) -> ("error out"=w462:errorcluster)  [unwired: 9 in, 1 out]
        n213 = Bundle By Name(cluster=w460, "StartMeas"=w456) -> (w459:T4)
        n214 = local write "Start"(w456) -> ()
        n215 = Build Array (concatenate)(w457, w458) -> (w455:T8[])
      }
      frame "GetResolution" {
        # "Resolution in ns"
        # "Gets resolution in ps"
        # "Resolution is saved in UIThread Data cluster in ns"
        n216 = Unbundle By Name(w468) -> ("DevIdx"=w470:i32)
        n217 = call "MH_GetResolution.vi"("devidx"=w470) -> ("error out"=w469:errorcluster, "resolution"=w466:dbl)  [unwired: 8 in, 1 out]
        n218 = Divide(x=w466, y=1000.0) -> (x/y=w464:dbl)
        n219 = Bundle By Name(cluster=w468, "Resolution"=w464) -> (w467:T4)
      }
      frame "GetAllHistos" {
        w501 = 1  # FLAG_OVERFLOW
        # "Provides a buffer (U32-array of length 'HistoLength' x nchannels) for all histograms."
        # "An alternative to GetHistos"
        n220 = Unbundle By Name(w488) -> ("Resolution"=w484:dbl, "DevIdx"=w492:i32, "HistoLength"=w495:i32, "Init Info.nchannels"=w496:i32, "max value"=w480:u32[], "CoincidenceArray"=w475:dbl[][])
        n221 = call "MH_AllocateAllHistoBuffer.vi"("NumChan"=w496, "HistoLength"=w495) -> ("Buffer"=w493:u32[])  [unwired: 9 in]
        n222 = call "MH_GetAllHistograms.vi"("Chcount"=w493, "devidx"=w492) -> ("error out"=w490:errorcluster, "Histograms"=w491:u32[])  [unwired: 7 in, 1 out]
        n223 = Reshape Array(w491, w496, w495) -> (w494:u32[][])
        n224 = call "MH_GetFlags.vi"("error in (no error)"=w490) -> ("error out"=w486:errorcluster, "flags"=w500:i32)  [unwired: 8 in, 1 out]
        n225 = And(x=w501, y=w500) -> (x .and. y?=w502:i32)
        n226 = Not Equal To 0?(x=w502) -> (x != 0?=→"OverFlow":bool)
        n227 = for {
          N: 4 -> [_]
          tunnel: [w521] -> w479 mode=indexing
          shift-right: [w523] -> w497
          shift-left: "Total Counts:\t\t" -> [w522]
          tunnel: w494 -> [w521] mode=indexing
          i -> [w527]
          n228 = Add Array Elements(numeric array=w521) -> (sum=w524:u32)
          n229 = Increment(x=w527) -> (x+1=w525:i32)
          n230 = Format Into String(format string="Ch.%2d: %d cnts.\t\t", initial string=w522, w525, w524) -> (resulting string=w523:string)  [unwired: 1 in, 1 out]
        }
        n231 = call "CalcRate.vi"("Refresh(ms)"="Refresh(ms)") -> ("Rate / Hz"=w478:dbl)  [unwired: 8 in, 2 out]
        n232 = Format Into String(format string="Readout Rate: %.1f Hz\\t\\t", w478) -> (resulting string=w506:string)  [unwired: 2 in, 1 out]
        n233 = for {
          tunnel: w484 -> [w516]
          tunnel: [w508] -> w476 mode=indexing
          tunnel: w480 -> [w515] mode=indexing
          tunnel: w479 -> [w512] mode=indexing
          tunnel: w478 -> [w511]
          tunnel: [w510] -> w477 mode=indexing
          n234 = Array Max & Min(array=w512) -> (max value=w510:u32, max index (indices)=w513:i32)  [unwired: 2 out]
          n235 = Subtract(x=w510, y=w515) -> (x-y=w514:u32)
          n236 = Multiply(x=w513, y=w516) -> (x*y=→"x*y":dbl)
          n237 = disable-structure shown="Enabled" {
            disable-tunnel: w514 -> [w519 w520]
            disable-tunnel: w511 -> [w518 _]
            disable-tunnel: [w517 w520] -> w508
            frame Disabled {
              n238 = Multiply(x=w519, y=w518) -> (x*y=w517:dbl)
            }
            frame Enabled {
            }
          }
        }
        n239 = Concatenate Strings(w506, w497) -> (w505:string)
        n240 = Bundle(0.0, "Resolution"=w484, "Histograms"=w479) -> (→"HistoGraph":T1)  [unwired: 1 in]
        n241 = local write "Status"(w505) -> ()
        n242 = Build Array (concatenate)(w475, w476) -> (w472:dbl[][])
        n243 = Send Notification(notification=w472, notifier=w482) -> (error out=w481:errorcluster)  [unwired: 1 in, 1 out]
        n244 = call "GetLastnElemsfromArray.vi"("array"=w472, "y"="Monitor Range") -> ("deleted portion"=w473:dbl[][])
        n245 = Merge Errors(w486, w481) -> (w485:errorcluster)
        n246 = Bundle By Name(cluster=w488, "max value"=w477, "CoincidenceArray"=w473) -> (w487:T4)
      }
      frame "GetHistos" {
        w538 = 1  # FLAG_OVERFLOW
        # "Provides a buffer (U32-array of length 'HistoLength') for histograms."
        # "An alternative to GetAllHistos"
        n247 = Unbundle By Name(w552) -> ("Resolution"=w549:dbl, "Init Info.nchannels"=w531:i32, "Channels"=w532:T3[], "DevIdx"=w551:i32, "HistoLength"=w550:i32)
        n248 = call "MH_AllocateHistoBuffer.vi"("HistoLength"=w550) -> ("Buffer"=w543:u32[])  [unwired: 10 in]
        n249 = for {
          N: w531 -> [_]
          tunnel: w551 -> [w565]
          tunnel: [w553] -> w541 mode=indexing
          tunnel: w543 -> [w563]
          shift-right: [w564] -> w540
          shift-left: errorcluster {"status"=FALSE, "code"=0, "source"=""} ("error IO") -> [w557]
          shift-right: [w558] -> w534
          shift-left: "Total Counts:\t\t" -> [w556]
          tunnel: w532 -> [w555] mode=indexing
          i -> [w562]
          n250 = Unbundle By Name(w555) -> ("Enable"=w554:bool)
          n251 = case shown="True" w554 {
            tunnel: w565 -> [_ w573]
            tunnel: [w566 w572] -> w564
            tunnel: w563 -> [w567 w571]
            tunnel: [w567 w570] -> w553
            tunnel: w562 -> [_ w569]
            tunnel: w557 -> [w566 w568]
            frame False {
            }
            frame True {
              n252 = call "MH_GetHistogram.vi"("Chcount"=w571, "error in (no error)"=w568, "channel"=w569, "devidx"=w573) -> ("error out"=w572:errorcluster, "Histogram"=w570:u32[])  [unwired: 5 in, 1 out]
            }
          }
          n253 = Add Array Elements(numeric array=w553) -> (sum=w559:u32)
          n254 = Increment(x=w562) -> (x+1=w560:i32)
          n255 = Format Into String(format string="Ch.%2d: %d cnts.\t\t", initial string=w556, w560, w559) -> (resulting string=w558:string)  [unwired: 1 in, 1 out]
        }
        n256 = call "CalcRate.vi"("Refresh(ms)"=u32 500) -> ("Rate / Hz"=w547:dbl)  [unwired: 8 in, 2 out]
        n257 = Format Into String(format string="Readout Rate: %.1f Hz\\t\\t", w547) -> (resulting string=w545:string)  [unwired: 2 in, 1 out]
        n258 = Concatenate Strings(w545, w534) -> (w544:string)
        n259 = Bundle(0.0, "Resolution"=w549, "Histogram"=w541) -> (w529:T14)  [unwired: 1 in]
        n260 = local write "HistoGraph"(w529) -> ()
        n261 = local write "Status"(w544) -> ()
        n262 = call "MH_GetFlags.vi"("error in (no error)"=w540) -> ("error out"=w548:errorcluster, "flags"=w537:i32)  [unwired: 8 in, 1 out]
        n263 = And(x=w538, y=w537) -> (x .and. y?=w539:i32)
        n264 = Not Equal To 0?(x=w539) -> (x != 0?=w530:bool)
        n265 = local write "OverFlow"(w530) -> ()
      }
      frame "WriteStatus" {
        n266 = Unbundle By Name(w576) -> ("Status"=→"Status":string)
      }
      frame "EnableControls" {
        n267 = property class="VI"() -> ("Panel"=w581:refnum<vi>)  [unwired: 2 in, 2 out]
        n268 = property class="Pnl"(reference=w581) -> ("Decos[]"=w582:refnum<vi>[])  [unwired: 1 in, 2 out]
        n269 = property class="Pnl"(reference=w581) -> ("Controls[]"=w580:refnum<vi>[])  [unwired: 1 in, 2 out]
        n270 = for {
          tunnel: w582 -> [w585] mode=indexing
          tunnel: TRUE -> [w584]
          n271 = property class="Decor"(reference=w585, "Visible"=w584) -> ()  [unwired: 1 in, 2 out]
        }
        n272 = for {
          tunnel: w580 -> [w588] mode=indexing
          tunnel: T9."Enabled" ("Disabled") -> [w587]
          tunnel: [w586] -> _
          n273 = property class="Ctl"(reference=w588, "DisabledEnum"=w587) -> (error out=w586:errorcluster)  [unwired: 1 in, 1 out]
        }
      }
      frame "DisableControls" {
        n274 = property class="VI"() -> ("Panel"=w593:refnum<vi>)  [unwired: 2 in, 2 out]
        n275 = property class="Pnl"(reference=w593) -> ("Decos[]"=w594:refnum<vi>[])  [unwired: 1 in, 2 out]
        n276 = property class="Pnl"(reference=w593) -> ("Controls[]"=w592:refnum<vi>[])  [unwired: 1 in, 2 out]
        n277 = for {
          tunnel: w594 -> [w597] mode=indexing
          tunnel: FALSE -> [w596]
          n278 = property class="Decor"(reference=w597, "Visible"=w596) -> ()  [unwired: 1 in, 2 out]
        }
        n279 = for {
          tunnel: w592 -> [w600] mode=indexing
          tunnel: T9."Disabled and Grayed Out" ("Disabled") -> [w599]
          tunnel: [w598] -> _
          n280 = property class="Ctl"(reference=w600, "DisabledEnum"=w599) -> (error out=w598:errorcluster)  [unwired: 1 in, 1 out]
        }
      }
      frame "Error" {
        w601 = T8[] [enum."Exit"] items=["Idle", "Init", "SetInpChan", "SetSyncDivider", "SetSyncTrg", "SetSyncOffset", "SetSyncDeadTime", "SetBinning", "SetHistoOffset", "SetHistoLen", "SetStopOvl", "SetBitShift", "SetHistoAcqTime", "GetRates", "GetAllRates", "StartMeas", "StopMeas", "AbortMeas", "GetResolution", "GetHistos", "GetAllHistos", "ReadFiFo", "WriteStatus", "Resize", "EnableControls", "DisableControls", "Error", "Exit", "Acquire", "InitAcquisition"]
        w604 = T15 1 items=["no dialog", "OK message", "continue or stop message", "OK message + warnings", "continue/stop + warnings"] ("type of dialog (OK msg:1)")
        # "Error case: If an error occures the user is informed and the programm terminates. Add your own code to handle error events (e.g. exception lists, etc.)"
        n281 = call <vilib>:"Simple Error Handler.vi"("type of dialog (OK msg:1)"=w604, "error in (no error)"=w603) -> ()  [unwired: 3 in, 5 out]
      }
      frame "Exit" {
        n282 = Unbundle By Name(w612) -> ("DevIdx"=w611:i32)
        n283 = call "MH_CloseDevice.vi"("devidx"=w611) -> ("error out"=w608:errorcluster)  [unwired: 9 in, 1 out]
        n284 = Release Notifier(notifier=w606, error in (no error)=w610) -> (error out=w609:errorcluster)  [unwired: 3 out]
        n285 = Merge Errors(w609, w608) -> (w607:errorcluster)
      }
      frame "Acquire" {
        w620 = T12 2 items=["HIST"=0, "T2"=2, "T3"=3] ("Mode")
        w623 = T8[] [enum."DisableControls", enum."Init"] items=["Idle", "Init", "SetInpChan", "SetSyncDivider", "SetSyncTrg", "SetSyncOffset", "SetSyncDeadTime", "SetBinning", "SetHistoOffset", "SetHistoLen", "SetStopOvl", "SetBitShift", "SetHistoAcqTime", "GetRates", "GetAllRates", "StartMeas", "StopMeas", "AbortMeas", "GetResolution", "GetHistos", "GetAllHistos", "ReadFiFo", "WriteStatus", "Resize", "EnableControls", "DisableControls", "Error", "Exit", "Acquire", "InitAcquisition"]
        n286 = Path To String(path="Path") -> (string=w617:string)
        n287 = call "python_acquisition_multiple_in_python.vi"("MH_UIThread_Data"=w615, "FileName"="FileName 2", "mode"=w620, "Number \nof Acquisitions"="Number of Acquisitions", "Directory"=w617) -> ("error out"=w616:errorcluster)  [unwired: 2 in]
        n288 = Build Array (concatenate)(w622, w623) -> (w614:T8[])
      }
      frame "InitAcquisition" {
        n289 = Unbundle By Name(w625) -> ("DevIdx"=w627:i32)
        n290 = call "MH_CloseDevice.vi"("devidx"=w627) -> ("error out"=w626:errorcluster)  [unwired: 9 in, 1 out]
        n291 = Build Array (concatenate)(w628, MH_UIThread_Cmds_T2."Acquire") -> (w624:T8[])
      }
    }
    n292 = call "MH_EnQErrorT2.vi"("error in (no error)"=w11, "Cmds_in"=w7) -> ("error out"=w10:errorcluster, "Array"=w9:T8[])  [unwired: 8 in]
  }
  n293 = while {
    tunnel: w2 -> [w632]
    stop <- w631 stop-if-true
    n294 = Wait on Notification(notifier=w632) -> (notification=→"Waveform Chart":dbl[][], error out=w631:errorcluster)  [unwired: 3 in, 2 out]
  }
